vi "init.vi"(8 "error in (no error)":errorcluster, 10 "Variant":variant, 11 "USB-6000 in":refnum<class "USB-6000.lvclass">) -> (0 "error out":errorcluster, 3 "USB-6000 out":refnum<class "USB-6000.lvclass">)   [LabVIEW 2025, in "USB IO.lvlib" / "USB-6000.lvclass"]
uses:
  USB-6000.lvclass
  USB-6000.lvclass/USB-6000.ctl
  <vilib>/DAQmx/create/channels.llb/DAQmx Create Channel (AI-Voltage-Basic).vi
  <vilib>/DAQmx/create/channels.llb/DAQmx Create Channel (DI-Digital Input).vi
  <vilib>/DAQmx/create/channels.llb/DAQmx Create Channel (DO-Digital Output).vi
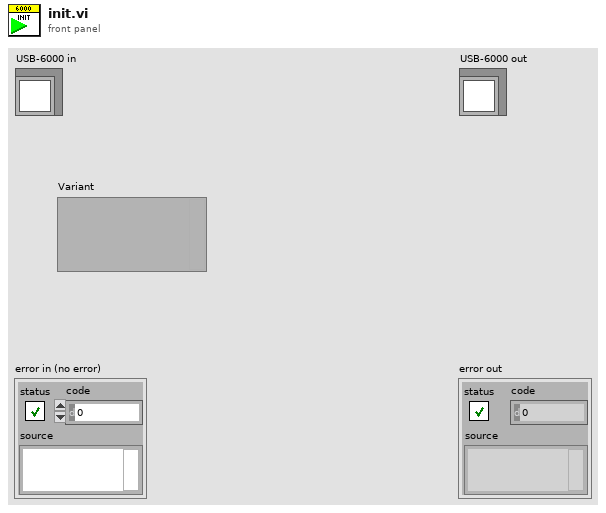
[diagram p1: front panel]
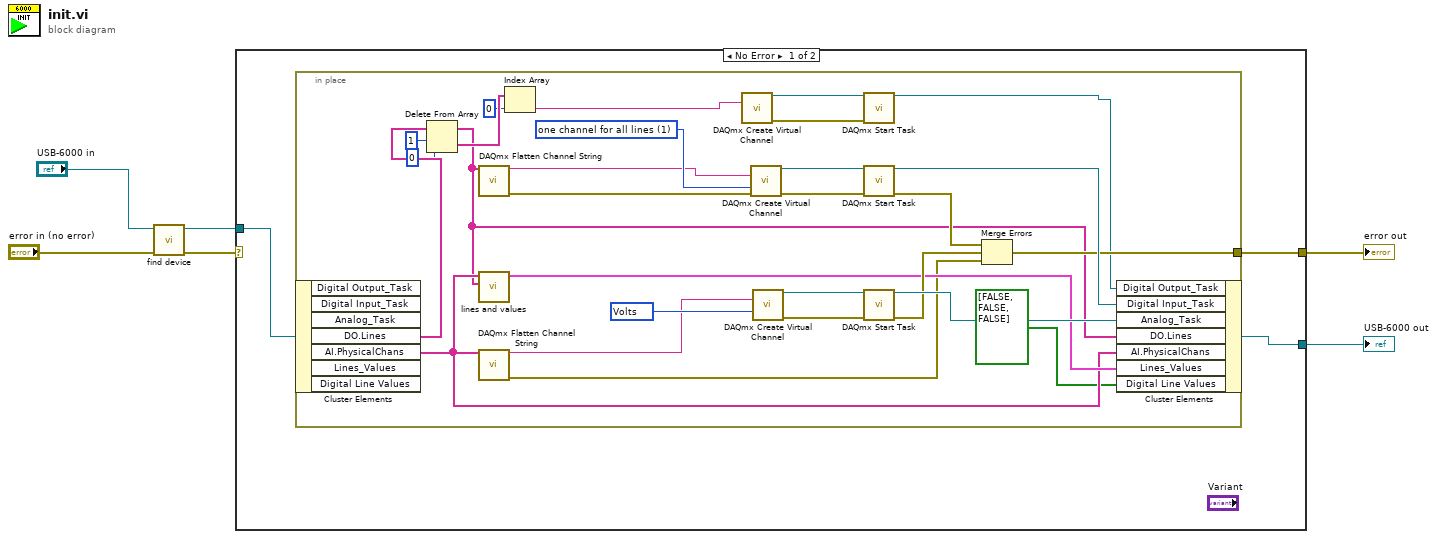
[diagram p0: block diagram]
diagram:
  n1 = call-dynamic "find device.vi"("error in (no error)"="error in (no error)", "USB-6000 in"="USB-6000 in") -> ("error out"=w2:errorcluster, "USB-6000 out"=w3:refnum<class "USB-6000.lvclass">)  [unwired: 8 in]
  n2 = case shown="No Error" w2 {
    selector: w2 -> [_ w39]
    tunnel: [w8 w39] -> w5
    tunnel: [w9 w38] -> w6
    tunnel: w3 -> [w7 w38]
    frame No Error {
      n3 = in-place {
        in-place-border: [w28] -> w8
        w26 = 10348 items=["Volts"=10348, "From Custom Scale"=10065] ("units")
        w37 = 1 items=["one channel for each line", "one channel for all lines"] ("line grouping")
        n4 = in-place-cluster #1(w7) -> ("DO.Lines"=w19:tag[], "AI.PhysicalChans"=w25:tag[])  [unwired: 5 out]
        n5 = Delete From Array(array=w19, length=1, index=0) -> (deleted portion=w16:tag[], array with subset deleted=w10:tag[])
        n6 = call <vilib>:"DAQmx Flatten Channel String.vi"("names in"=w10) -> ("names out"=w21:string, "error out"=w20:errorcluster)  [unwired: 13 in]
        n7 = call "lines and values.vi"("DO.Lines"=w10, "AI.PhysicalChans"=w25) -> ("Array"=w27:cluster{"Line":string, "Value":i32}[])  [unwired: 9 in]
        n8 = call <vilib>:"DAQmx Flatten Channel String.vi"("names in"=w25) -> ("names out"=w24:string, "error out"=w23:errorcluster)  [unwired: 13 in]
        n9 = Index Array(array=w16, index=0) -> (element=w14:tag)
        n10 = call-poly <vilib>:"DAQmx Create Virtual Channel.vi"("lines"=w14) -> ("task out"=w12:refnum<k21>, "error out"=w13:errorcluster)  [unwired: 13 in]
        n11 = call-poly <vilib>:"DAQmx Create Virtual Channel.vi"("lines"=w21, "line grouping"=w37, "error in"=w20) -> ("task out"=w36:refnum<k21>, "error out"=w35:errorcluster)  [unwired: 11 in]
        n12 = call-poly <vilib>:"DAQmx Create Virtual Channel.vi"("physical channels"=w24, "units"=w26) -> ("task out"=w34:refnum<k21>, "error out"=w33:errorcluster)  [unwired: 12 in]
        n13 = call <vilib>:"DAQmx Start Task.vi"("task/channels in"=w12, "error in"=w13) -> ("task out"=w11:refnum<k21>)  [unwired: 12 in, 1 out]
        n14 = call <vilib>:"DAQmx Start Task.vi"("task/channels in"=w36, "error in"=w35) -> ("task out"=w31:refnum<k21>, "error out"=w29:errorcluster)  [unwired: 12 in]
        n15 = call <vilib>:"DAQmx Start Task.vi"("task/channels in"=w34, "error in"=w33) -> ("task out"=w32:refnum<k21>, "error out"=w30:errorcluster)  [unwired: 12 in]
        n16 = Merge Errors(w29, w30, w23) -> (w28:errorcluster)
        n17 = in-place-cluster #1("Digital Output_Task"=w11, "Digital Input_Task"=w31, "Analog_Task"=w32, "DO.Lines"=w10, "AI.PhysicalChans"=w25, "Lines_Values"=w27, "Digital Line Values"=bool[] [FALSE, FALSE, FALSE]) -> (w9:refnum<class "USB-6000.lvclass">)
      }
    }
    frame Error {
    }
  }
  "error out" <- w5
  "USB-6000 out" <- w6
